vi "BotSpeak.InitQueue.vi"() -> (0 "ReadQueue":refnum<queue>, 1 "SendQueue":refnum<queue>)   [LabVIEW 2014]
uses:
  <userlib>/botspeak/VIs/Direct/BotSpeak_Control.ctl
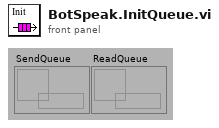
[diagram p1: front panel]
types:
  T1 = typedef "BotSpeak_Control.ctl" = cluster{"Address":string, "Reply EOF":string, "Hardware":string, "Retries":i8, "Timeout":i32, "Open?":bool}
  T2 = cluster{"Bot Settings":T1, "String":string, "ID":dbl, "Caller":string}
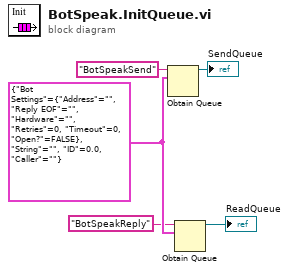
[diagram p0: block diagram]
diagram:
  w5 = T2 {"Bot Settings"={"Address"="", "Reply EOF"="", "Hardware"="", "Retries"=0, "Timeout"=0, "Open?"=FALSE}, "String"="", "ID"=0.0, "Caller"=""}
  n1 = Obtain Queue(name (unnamed)="BotSpeakSend", element data type=w5) -> (queue out=→"SendQueue":refnum<queue>)  [unwired: 3 in, 2 out]
  n2 = Obtain Queue(name (unnamed)="BotSpeakReply", element data type=w5) -> (queue out=→"ReadQueue":refnum<queue>)  [unwired: 3 in, 2 out]
